vi "Get value.vi"(8 "error in (no error)":errorcluster, 11 "Stack in":refnum<class "Stack.lvclass">) -> (0 "error out":errorcluster, 2 "Value":dbl, 3 "Stack out":refnum<class "Stack.lvclass">)   [LabVIEW 2021, in "Stack.lvclass"]
uses:
  Stack.lvclass
  Stack.lvclass/Stack.ctl
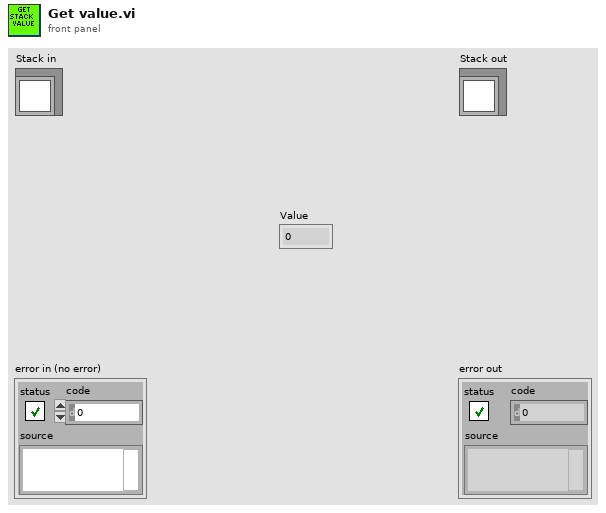
[diagram p1: front panel]
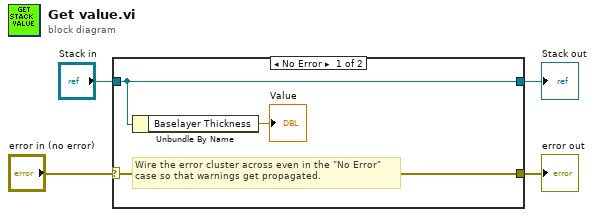
[diagram p0: block diagram]
diagram:
  n1 = case shown="No Error" "error in (no error)" {
    selector: "error in (no error)" -> [w7 w9]
    tunnel: [w7 w9] -> w3
    tunnel: [w5 w8] -> w1
    tunnel: "Stack in" -> [w5 w8]
    frame No Error {
      # "Wire the error cluster across even in the \"No Error\"\ncase so that warnings get propagated."
      n2 = Unbundle By Name(w5) -> ("Baselayer Thickness"=→"Value":dbl)
    }
    frame Error {
    }
  }
  "error out" <- w3
  "Stack out" <- w1
